vi "TSM Set DAQmx AO Tasks.vi"(0 "TSM context":T1, 1 "IdleOutputBehavior (Zero Volts)":i32(ring)=12526 items=["Zero Volts"=12526, "High-Impedance"=12527, "Maintain Existing Value"=12528], 5 "Sampling Rate (Hz)":dbl format="%#_6pHz", 7 "Samples per channel":i32=1000, 9 "Range (V)":dbl=5.0 format="%#_13g", 11 "error in (no error)":errorcluster) -> (15 "error out":errorcluster)   [LabVIEW 2020]
doc: "Use this VI to initialize AI and AO tasks for all NI-DAQmx instruments in the pin map associated with the test program."
uses:
  <vilib>/NI_TestStand_SemiconductorModule/NI_TestStand_Semiconductor_Module.lvlibp/PinMap/General/SemiconductorModuleContext.ctl
  <vilib>/DAQmx/create/channels.llb/DAQmx Create Channel (AO-Voltage-Basic).vi
  <vilib>/DAQmx/configure/timing.llb/DAQmx Timing (Sample Clock).vi
  <vilib>/NI_TestStand_SemiconductorModule/NI_TestStand_Semiconductor_Module.lvlibp
  <resource>/objmgr/daqmx.rc
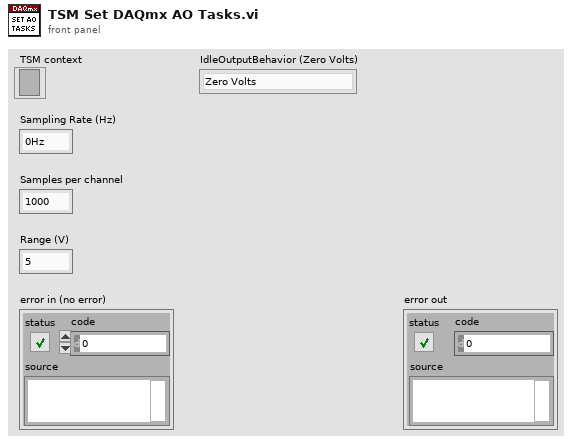
[diagram p1: front panel]
types:
  T1 = typedef "NI_TestStand_Semiconductor_Module.lvlibp/SemiconductorModuleContext.ctl" = refnum<k7>
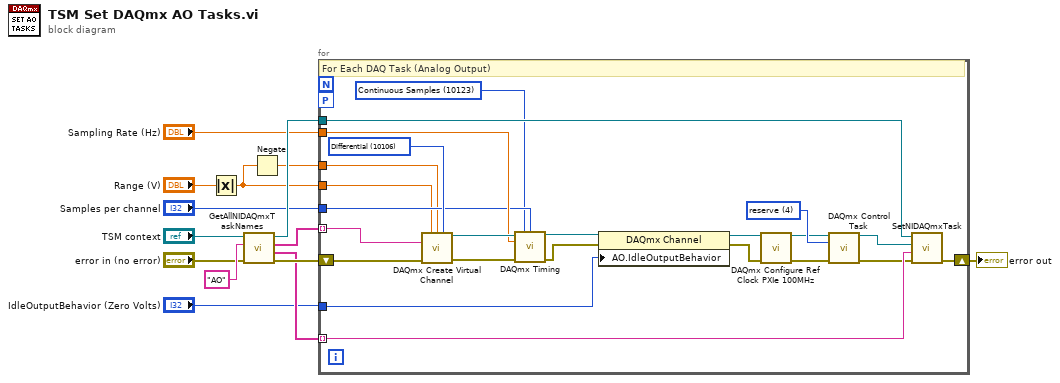
[diagram p0: block diagram]
diagram:
  n1 = Absolute Value(x="Range (V)") -> (abs(x)=w3:dbl)
  n2 = call <vilib>:"GetAllNIDAQmxTaskNames.vi"("error in (no error)"="error in (no error)", "Task Type"="AO", "Semiconductor Module Context"="TSM context") -> ("error out"=w13:errorcluster, "Task Names"=w12:string[], "Channel Lists"=w11:string[], "Semiconductor Module Context Out"=w14:T1)  [unwired: 5 in]
  n3 = Negate(x=w3) -> (-x=w2:dbl)
  n4 = for {
    tunnel: w14 -> [w36]
    tunnel: w12 -> [w32] mode=indexing
    tunnel: w11 -> [w34] mode=indexing
    shift-right: [w35] -> w6
    shift-left: w13 -> [w37]
    tunnel: "Sampling Rate (Hz)" -> [w29]
    tunnel: "Samples per channel" -> [w28]
    tunnel: "IdleOutputBehavior (Zero Volts)" -> [w21]
    workers-P: _ -> [_]
    tunnel: w3 -> [w20]
    tunnel: w2 -> [w15]
    w26 = 4 items=["verify"=2, "reserve"=4, "commit"=3, "unreserve"=5, "abort"=6] ("action")
    w27 = 10123 items=["Finite Samples"=10178, "Continuous Samples"=10123, "Hardware Timed Single Point"=12522] ("sample mode")
    w33 = 10106 items=["default"=-1, "RSE"=10083, "NRSE"=10078, "Differential"=10106, "Pseudodifferential"=12529] ("input terminal configuration")
    # "For Each DAQ Task (Analog Output)"
    n5 = call-poly <vilib>:"DAQmx Create Virtual Channel.vi"("maximum value"=w20, "minimum value"=w15, "output terminal configuration"=w33, "physical channels"=w34, "error in"=w37) -> ("task out"=w30:refnum<k21>, "error out"=w31:errorcluster)  [unwired: 9 in]
    n6 = call-poly <vilib>:"DAQmx Timing.vi"("task/channels in"=w30, "sample mode"=w27, "samples per channel"=w28, "rate"=w29, "error in"=w31) -> ("task out"=w23:refnum<k21>, "error out"=w22:errorcluster)  [unwired: 9 in]
    n7 = property class="DAQmx Channel"(reference=w23, error in=w22, "AO.IdleOutputBehavior"=w21) -> (reference out=w19:refnum<k21>, error out=w18:errorcluster)
    n8 = call "DAQmx Configure Ref Clock PXIe 100MHz.vi"("DAQmx Task In"=w19, "error in (no error)"=w18) -> ("DAQmx Task Out"=w17:refnum<k21>, "error out"=w16:errorcluster)  [unwired: 12 in]
    n9 = call <vilib>:"DAQmx Control Task.vi"("task/channels in"=w17, "action"=w26, "error in"=w16) -> ("task out"=w25:refnum<k21>, "error out"=w24:errorcluster)  [unwired: 11 in]
    n10 = call <vilib>:"SetNIDAQmxTask.vi"("error in (no error)"=w24, "Task Name"=w32, "DAQmx Task"=w25, "Semiconductor Module Context"=w36) -> ("error out"=w35:errorcluster)  [unwired: 6 in, 1 out]
  }
  "error out" <- w6
